vi "ECAT Start FoE Write.vi"(8 "error in":errorcluster, 9 "Device Filename":string, 11 "Slave Ref in":refnum<k21>) -> (0 "error out":errorcluster, 3 "Slave Ref out":refnum<k21>)   [LabVIEW 2011, in "Scan Engine Custom Device.lvlib"]
uses:
  Scan Engine Custom Device.lvlib
  Program Files (x86)/National Instruments/LabVIEW 2011/resource/objmgr/IndComECAT.rc
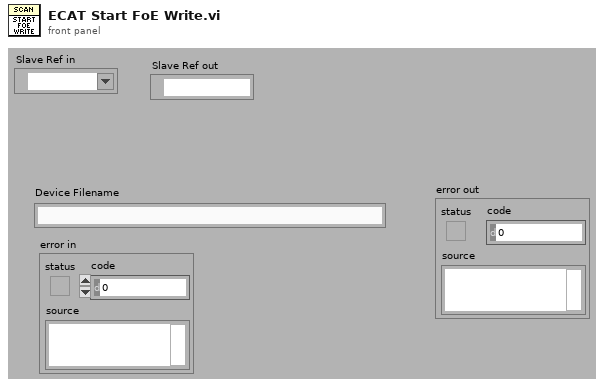
[diagram p1: front panel]
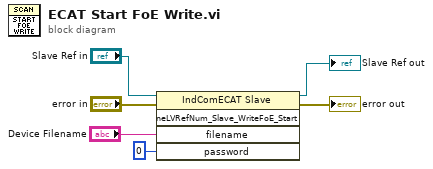
[diagram p0: block diagram]
diagram:
  n1 = invoke class="IndComECAT Slave" method="neLVRefNum_Slave_WriteFoE_Start"(reference="Slave Ref in", error in="error in", "filename"="Device Filename", "password"=u32 0) -> (reference out=→"Slave Ref out":refnum<k21>, error out=→"error out":errorcluster)  [unwired: 1 in, 3 out]
